vi "Test Traduction.vi"() -> ()   [LabVIEW 2013]
uses:
  <vilib>/Utility/miscctls.llb/LVPointTypeDef.ctl
panel:
  in  "stop":bool caption="Arrêter"
  in  "Langues":u16(ring)=1 caption="Choose" items=["Français", "English"]
  in  "Traduction 2D [ ]":string[][](array[string])=[["Configuration Caption", "Français", "Anglais"], ["Type FC", "Type@@@unique;empilement;", "Type@@@one;stack;"], ["Surface", "Surface (cm2)", "Area (cm2)"], ["Nbre cellules", "cellules", "Cells"], ["Tab Paramètres&Température&T Essai affiché", "Températures visées (°C):", "Temperatures Set Point (°C):"], ["Tab Paramètres&Température&T Essai affiché&Bouteille eau H2", "Bouteille eau H2", "Water Bottle H2"], ["Tab Paramètres&Température&T Essai affiché&Ligne H2", "Ligne H2", "H2 Line"], ["Tab Paramètres&Température&T Essai affiché&Bouteille eau O2 ", "Bouteille eau O2 ", "Water Bottle O2"], ["Tab Paramètres&Température&T Essai affiché&Ligne O2", "Ligne O2", "O2 Line"], ["Tab Paramètres&Température&T Essai affiché&Température pile à combustible", "Pile à combustible", "Fuel Cell"], ["Tab Paramètres&Charge électronique&Mode de polarisation", "Mode de polarisation@@@Courant constant;Voltage constant;Puissance constante;Résistance constante;", "Polarization Mode@@@Constant Current;Constant Voltage;Constant Power;Constant Resistance;"], ["Tab Paramètres&Charge électronique&Balayage au début ", "Courbe de polarisation au début?", "Polarization Curve at Start?"], ["Tab Paramètres", "Températures;Gas;Charge électronique;", "Temperatures;Gaz;Electronic Load;"], ["Tab Paramètres&Charge électronique&Choisir cycle activation", "Choisir;", "Choose;"], ["TitreVIConfiguration", "Essai traduction...", "Test Traduction..."], ["Titre", "@@@Français", "@@@English"], ["stop", ";Arrêter", ";Stop"], ["Langues", "Choisir@@@Français;English;", "Choose@@@Français;English;"]]
  out "Control references [ ]":T1(array[cluster])=[{"Nom"="Titre", "Label ?"=FALSE, "Caption ?"=FALSE, "Ref"=refnum}, {"Nom"="Langues", "Label ?"=FALSE, "Caption ?"=TRUE, "Ref"=refnum}, {"Nom"="Type FC", "Label ?"=FALSE, "Caption ?"=TRUE, "Ref"=refnum}, {"Nom"="Nbre cellules", "Label ?"=FALSE, "Caption ?"=TRUE, "Ref"=refnum}, {"Nom"="Surface", "Label ?"=FALSE, "Caption ?"=TRUE, "Ref"=refnum}, {"Nom"="Tab Paramètres", "Label ?"=FALSE, "Caption ?"=FALSE, "Ref"=refnum}, {"Nom"="Tab Paramètres&Température&T Essai affiché", "Label ?"=FALSE, "Caption ?"=TRUE, "Ref"=refnum}, {"Nom"="Tab Paramètres&Température&T Essai affiché&Bouteille eau H2", "Label ?"=FALSE, "Caption ?"=TRUE, "Ref"=refnum}, {"Nom"="Tab Paramètres&Température&T Essai affiché&Ligne H2", "Label ?"=FALSE, "Caption ?"=TRUE, "Ref"=refnum}, {"Nom"="Tab Paramètres&Température&T Essai affiché&Bouteille eau O2 ", "Label ?"=FALSE, "Caption ?"=TRUE, "Ref"=refnum}, {"Nom"="Tab Paramètres&Température&T Essai affiché&Ligne O2", "Label ?"=FALSE, "Caption ?"=TRUE, "Ref"=refnum}, {"Nom"="Tab Paramètres&Température&T Essai affiché&Température pile à combustible", "Label ?"=FALSE, "Caption ?"=TRUE, "Ref"=refnum}, {"Nom"="Tab Paramètres&Charge électronique&Choisir cycle activation", "Label ?"=FALSE, "Caption ?"=TRUE, "Ref"=refnum}, {"Nom"="Tab Paramètres&Charge électronique&Mode de polarisation", "Label ?"=FALSE, "Caption ?"=TRUE, "Ref"=refnum}, {"Nom"="Tab Paramètres&Charge électronique&Balayage au début ", "Label ?"=FALSE, "Caption ?"=TRUE, "Ref"=refnum}, {"Nom"="stop", "Label ?"=FALSE, "Caption ?"=FALSE, "Ref"=refnum}]
  in  "Type FC":i16(ring)=1 caption="Type" items=["one", "stack"]
  in  "Surface":sgl=1.0 caption="Area (cm2)" min=0 format="%#.3f"
  in  "Nbre cellules":u16=1 caption="Cells" min=1 step=1
  in  "Tab Paramètres":T2(tab)=enum."Gas"
  in  "T Essai affiché":T3 caption="Temperatures Set Point (°C):" {"Température pile à combustible" min=0.0 max=200.0; "Ligne O2" min=0.0 max=200.0; "Bouteille eau O2" min=0.0 max=200.0; "Ligne H2" min=0.0 max=200.0; "Bouteille eau H2" min=0.0 max=200.0}
  in  "Choisir cycle activation":bool caption="Choose"
  in  "Mode de polarisation":i16(ring)=3 caption="Polarization Mode" items=["Constant Current", "Constant Voltage", "Constant Power", "Constant Resistance"]
  in  "Balayage au début":bool=TRUE caption="Polarization Curve at Start?"
  out "Titre":string="English"
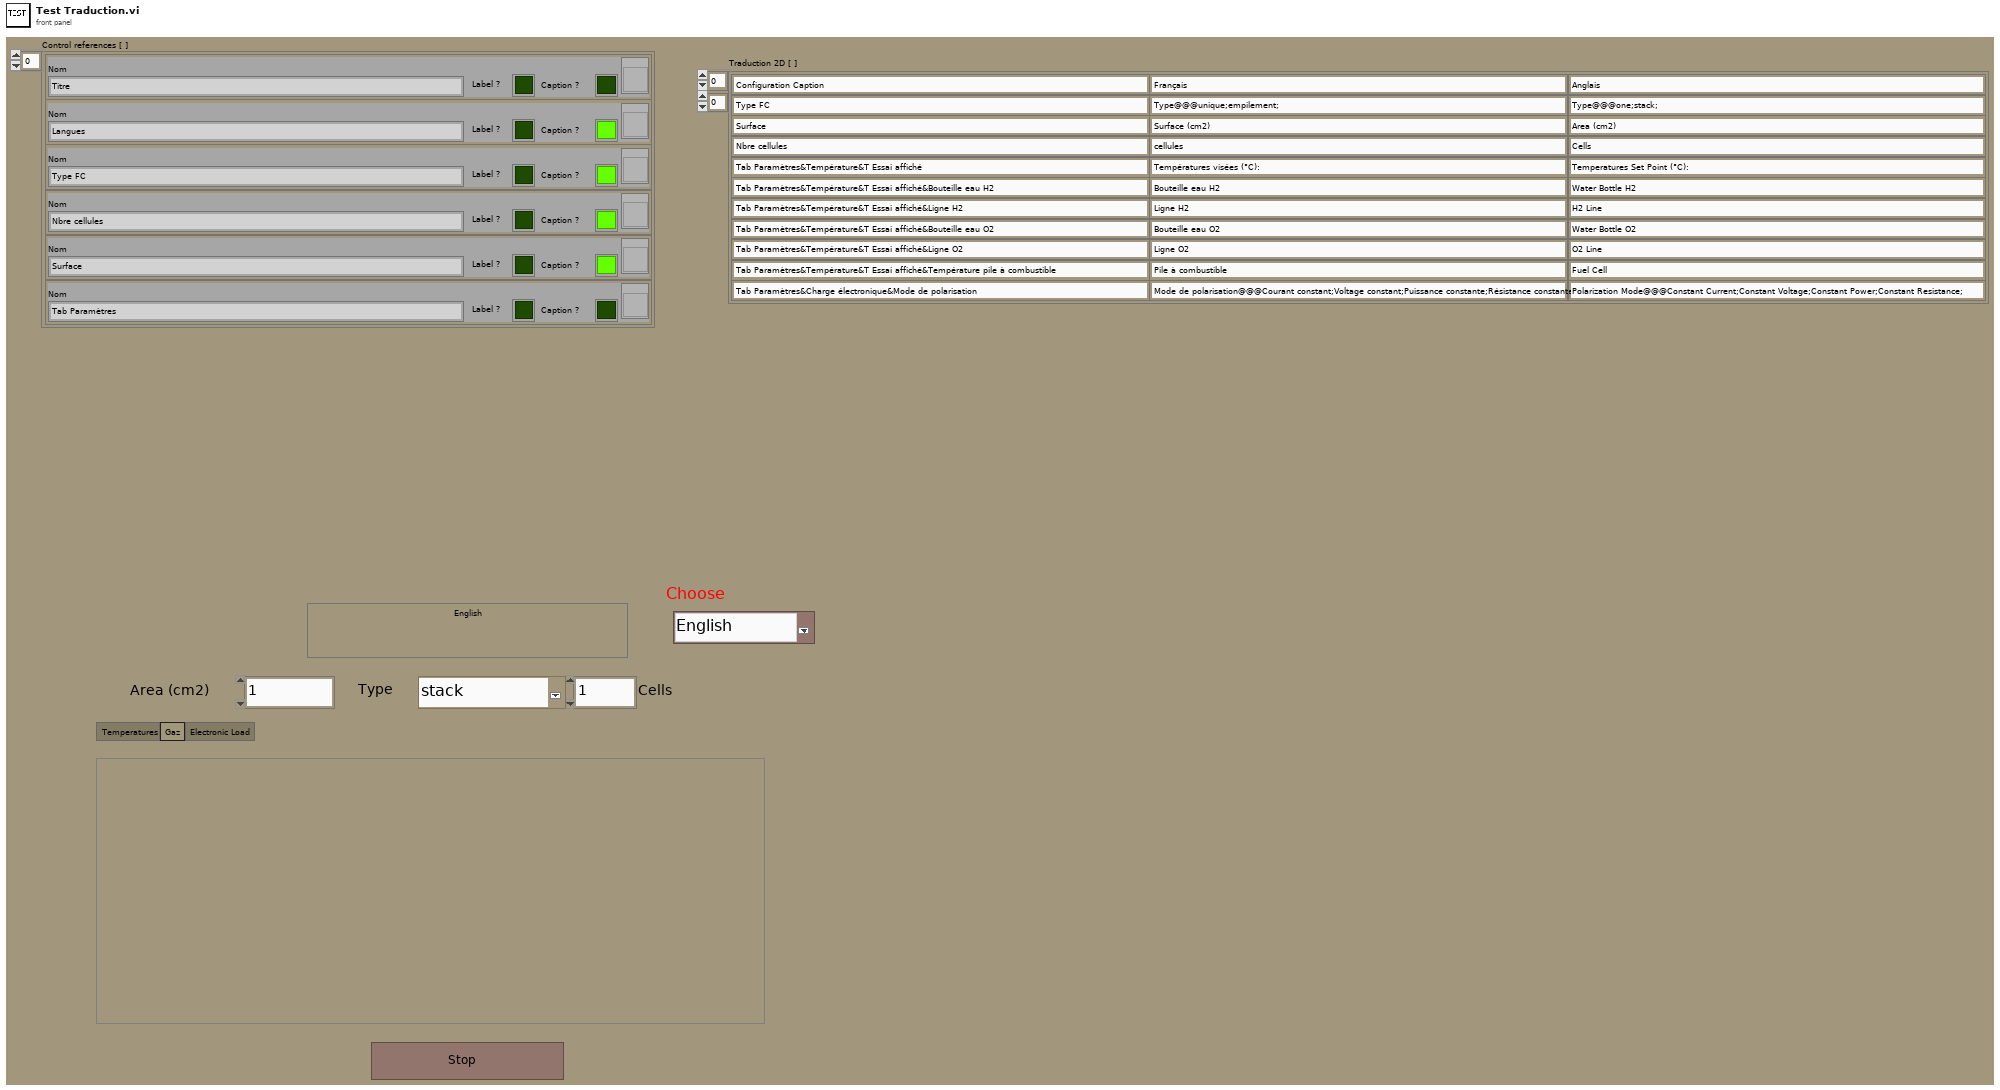
[diagram p1: front panel]
types:
  T1 = cluster{"Nom":string, "Label ?":bool, "Caption ?":bool, "Ref":refnum<vi>}[]
  T2 = enum32{"Température", "Gas", "Charge électronique", "Ancien essai"}
  T3 = cluster{"Bouteille eau H2":dbl, "Ligne H2":dbl, "Bouteille eau O2 ":dbl, "Ligne O2":dbl, "Température pile à combustible":dbl}
  T4 = typedef "LVPointTypeDef.ctl" = cluster{"Horizontal":i16, "Vertical":i16}
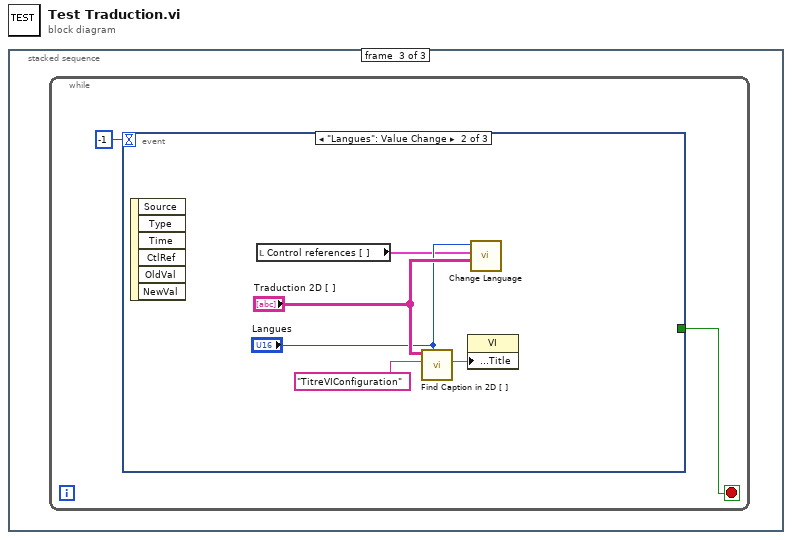
[diagram p0: block diagram]
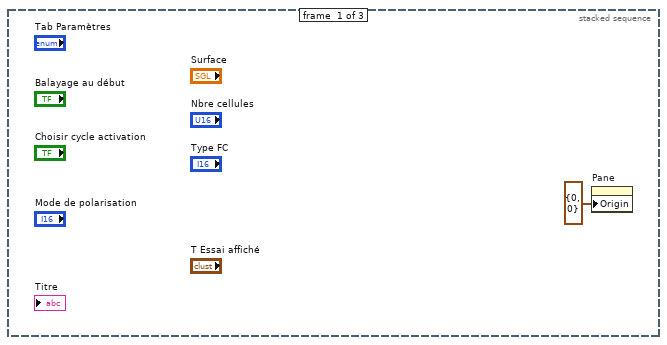
[diagram p2: hidden frame]
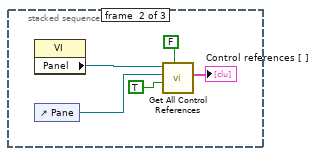
[diagram p3: hidden frame]
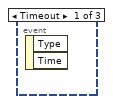
[diagram p4: hidden frame]
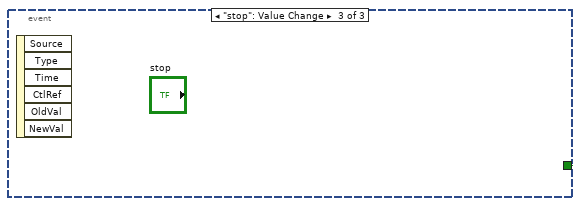
[diagram p5: hidden frame]
diagram:
  n1 = stacked-sequence {
    frame #0 {
      n2 = property on="Pane" class="Pane"("Origin"=T4 {"Horizontal"=0, "Vertical"=0}) -> ()  [unwired: 2 in, 2 out]
    }
    frame #1 {
      n3 = property class="VI"() -> ("Panel"=w4:refnum<vi>)  [unwired: 2 in, 2 out]
      n4 = control-ref of="Pane"() -> (w3:refnum<vi>)
      n5 = call "Get All Control References.vi"("Label seulement"=FALSE, "In the pane"=TRUE, "Pane refnum"=w3, "Panel refnum"=w4) -> ("Control references [ ]"=→"Control references [ ]":T1)  [unwired: 1 in, 4 out]
    }
    frame #2 {
      n6 = while {
        stop <- w7 stop-if-true
        n7 = event shown="[1] \"Langues\": Value Change" {
          selector: _ -> [_ _ _]
          dyn-events: _ -> [_ _ _]
          timeout: -1 -> [_ _ _]
          tunnel: [_ _ TRUE] -> w7
          event Timeout {
            n8 = event-data() -> ()  [unwired: 3 out]
          }
          event "Langues": Value Change {
            n9 = event-data() -> ()  [unwired: 7 out]
            n10 = local read "Control references [ ]"() -> (w9:T1)
            n11 = call "Find Caption in 2D [ ].vi"("Langues/Languages"="Langues", "Nom"="TitreVIConfiguration", "Array IN"="Traduction 2D [ ]") -> ("Légende"=w13:string)  [unwired: 2 in, 6 out]
            n12 = property class="VI"("Front Panel.Title"=w13) -> ()  [unwired: 2 in, 2 out]
            n13 = call "Change Language.vi"("Array IN"="Traduction 2D [ ]", "References Pane"=w9, "Langues/Languages"="Langues") -> ()  [unwired: 9 out]
          }
          event "stop": Value Change {
            n14 = event-data() -> ()  [unwired: 7 out]
          }
        }
      }
    }
  }
